vi "Get Medio data average.vi"(9 "precision (6)":i16=3, 11 "Waveform Graph":dbl[](graph)) -> (3 "mean":dbl format="%0.6f")   [LabVIEW 2021]
uses:
  <vilib>/Analysis/NI_AALBase.lvlib
  <vilib>/Analysis/baseanly.llb/Mean (DBL).vi
panel:
  in  "length":i32=30
  out "median 2":dbl format="%0.3f"
  out "median":dbl format="%0.2f"
  out "Waveform Graph 3":dbl[](graph)
  out "Waveform Graph 2":dbl[](graph)
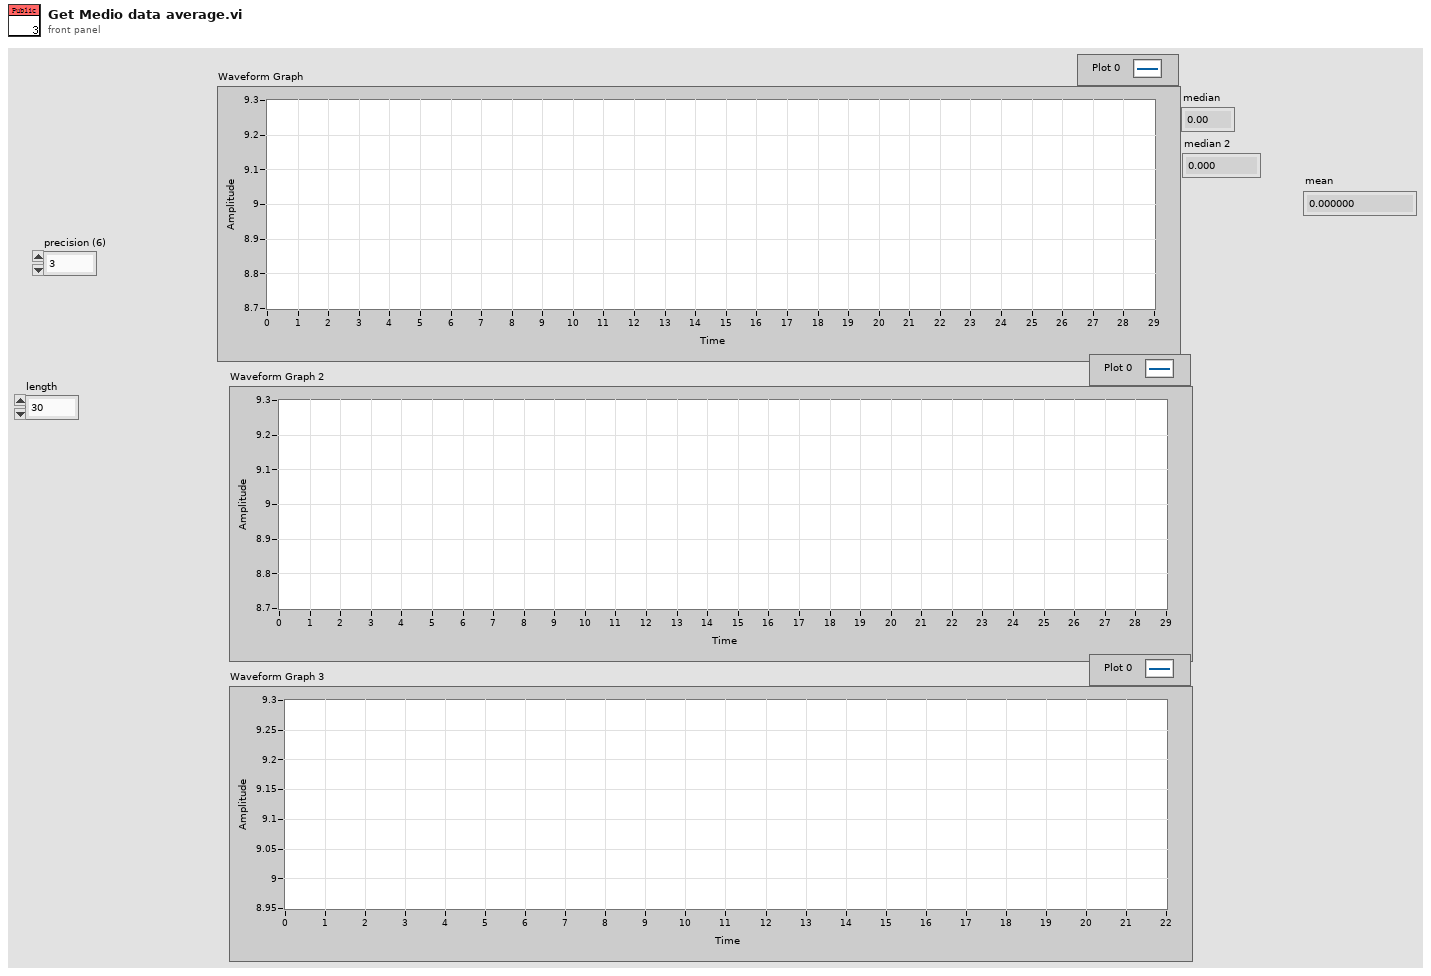
[diagram p1: front panel]
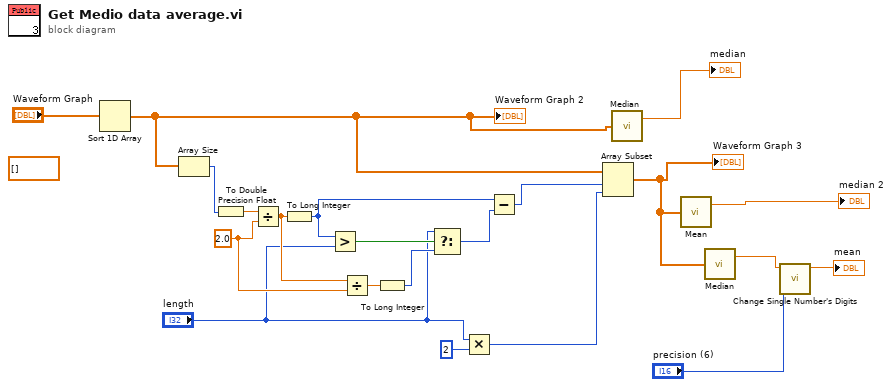
[diagram p0: block diagram]
diagram:
  w12 = 2.0 ("y")
  (unwired) dbl[] [] ("Waveform Graph")
  n1 = Sort 1D Array(array="Waveform Graph") -> (sorted array=w9:dbl[])
  "Waveform Graph 2" <- w9
  n2 = Array Size(array=w9) -> (size(s)=w20:i32)
  n3 = To Double Precision Float(number=w20) -> (double precision float=w19:dbl)
  n4 = Divide(x=w19, y=w12) -> (x/y=w18:dbl)
  n5 = To Long Integer(number=w18) -> (32bit integer=w16:i32)
  n6 = Greater?(x=w16, y="length") -> (0:w17:bool)
  n7 = Divide(x=w18, y=w12) -> (x/y=w15:dbl)
  n8 = To Long Integer(number=w15) -> (32bit integer=w14:i32)
  n9 = Select(t="length", s=w17, f=w14) -> (s? t:f=w11:i32)
  n10 = Multiply(x="length", y=2) -> (x*y=w1:i32)
  n11 = Subtract(x=w16, y=w11) -> (x-y=w13:i32)
  n12 = Array Subset(array=w9, index=w13, length=w1) -> (w10:dbl[])
  "Waveform Graph 3" <- w10
  n13 = call <vilib>:"Median.vi"("X"=w9) -> ("median"=→"median":dbl)  [unwired: 1 out]
  n14 = call-poly <vilib>:"Mean.vi"("X"=w10) -> ("mean"=→"median 2":dbl)  [unwired: 1 out]
  n15 = call <vilib>:"Median.vi"("X"=w10) -> ("median"=w6:dbl)  [unwired: 1 out]
  n16 = call <userlib>:"Change Single Number's Digits.vi"("precision (6)"="precision (6)", "number"=w6) -> ("number 2"=→"mean":dbl)  [unwired: 8 in, 1 out]
